vi "WCA_Global.vi"() -> ()   [LabVIEW 2017]
panel:
  out "Link":bool
  out "Slave Node in":cluster{"Address":i16, "Serial Number":i8[]} {"Serial Number" format="%.0x"; "Address" format="%.0x"}
  out "ObjHandle out":u32
  # "Node Address"
  # "Serial Number"
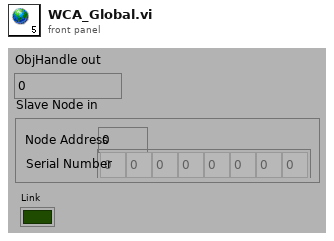
[diagram p1: front panel]
diagram:
